vi "ColorsTable.vi"(11 "2D String":string[][](array[string])) -> (0 "Table":string[][](table))   [LabVIEW 2023]
panel:
  in  "Sorted":bool
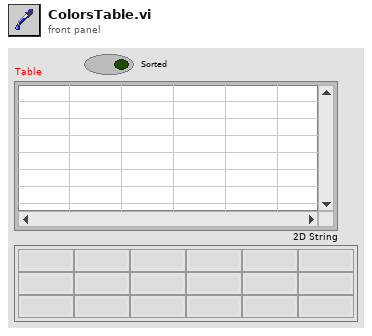
[diagram p1: front panel]
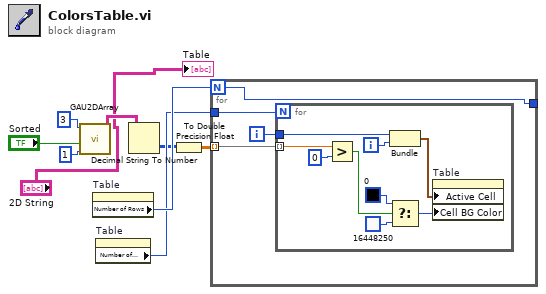
[diagram p0: block diagram]
diagram:
  n1 = call "GAU2DArray.vi"("Colums"=1, "Sorted"="Sorted", "Rows"=3) -> ("2D String Array"=w2:string[][])  [unwired: 6 in, 2 out]
  n2 = property on="Table" class="Tbl (strict)"() -> ("Number of Rows"=w6:u32)  [unwired: 2 in, 2 out]
  n3 = property on="Table" class="Tbl (strict)"() -> ("Number of Columns"=w5:u32)  [unwired: 2 in, 2 out]
  n4 = Decimal String To Number(string=w2) -> (number=w4:i32[][])  [unwired: 2 in, 1 out]
  n5 = To Double Precision Float(number=w4) -> (double precision float=w3:dbl[][])
  n6 = for {
    N: w6 -> [w11]
    tunnel: w5 -> [w13]
    tunnel: w3 -> [w12] mode=indexing
    tunnel: [w11] -> _
    i -> [w10]
    n7 = for {
      N: w13 -> [_]
      tunnel: w12 -> [w22] mode=indexing
      tunnel: w10 -> [w20]
      i -> [w19]
      n8 = Greater?(x=w22, y=0) -> (0:w17:bool)
      n9 = Bundle(w20, w19) -> (w18:cluster{i32, i32})  [unwired: 1 in]
      n10 = Select(t=u32 0 ("Active Cell:Cell Background Color"), s=w17, f=u32 16448250 ("Active Cell:Cell Background Color")) -> (s? t:f=w14:u32)
      n11 = property on="Table" class="Tbl (strict)"("Active Cell"=w18, "Cell BG Color"=w14) -> ()  [unwired: 2 in, 2 out]
    }
  }
  "Table" <- "2D String"
